vi "frontPanel.vi"(8 "error in (no error)":errorcluster, 10 "closeViewerEvent":refnum<user-event>, 11 "AnalysisResultsViewer in":refnum<class "AnalysisResultsViewer.lvclass">) -> (0 "error out":errorcluster, 3 "AnalysisResultsViewer out":refnum<class "AnalysisResultsViewer.lvclass">)   [LabVIEW 2009, in "Views.lvlib" / "Camera.lvlib" / "AnalysisResultsViewer.lvclass"]
uses:
  AnalysisResultsViewer.lvclass
  AnalysisResultsViewer.lvclass/AnalysisResultsViewer.ctl
panel:
  in  "timescale":dbl=1000.0
  in  "ResultsBox":i32(listbox)
  out "Cloud Size y":dbl(graph)
  in  "stop":bool
  out "Cloud Size x":dbl(graph)
  out "Atom Number":dbl(graph)
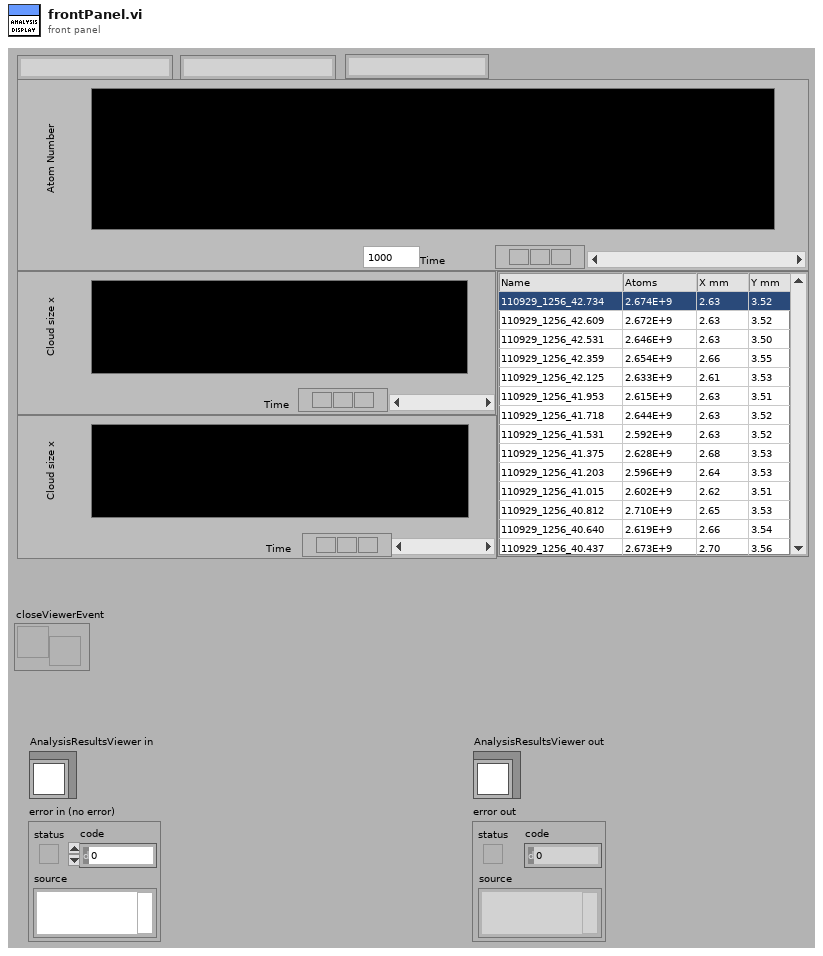
[diagram p1: front panel]
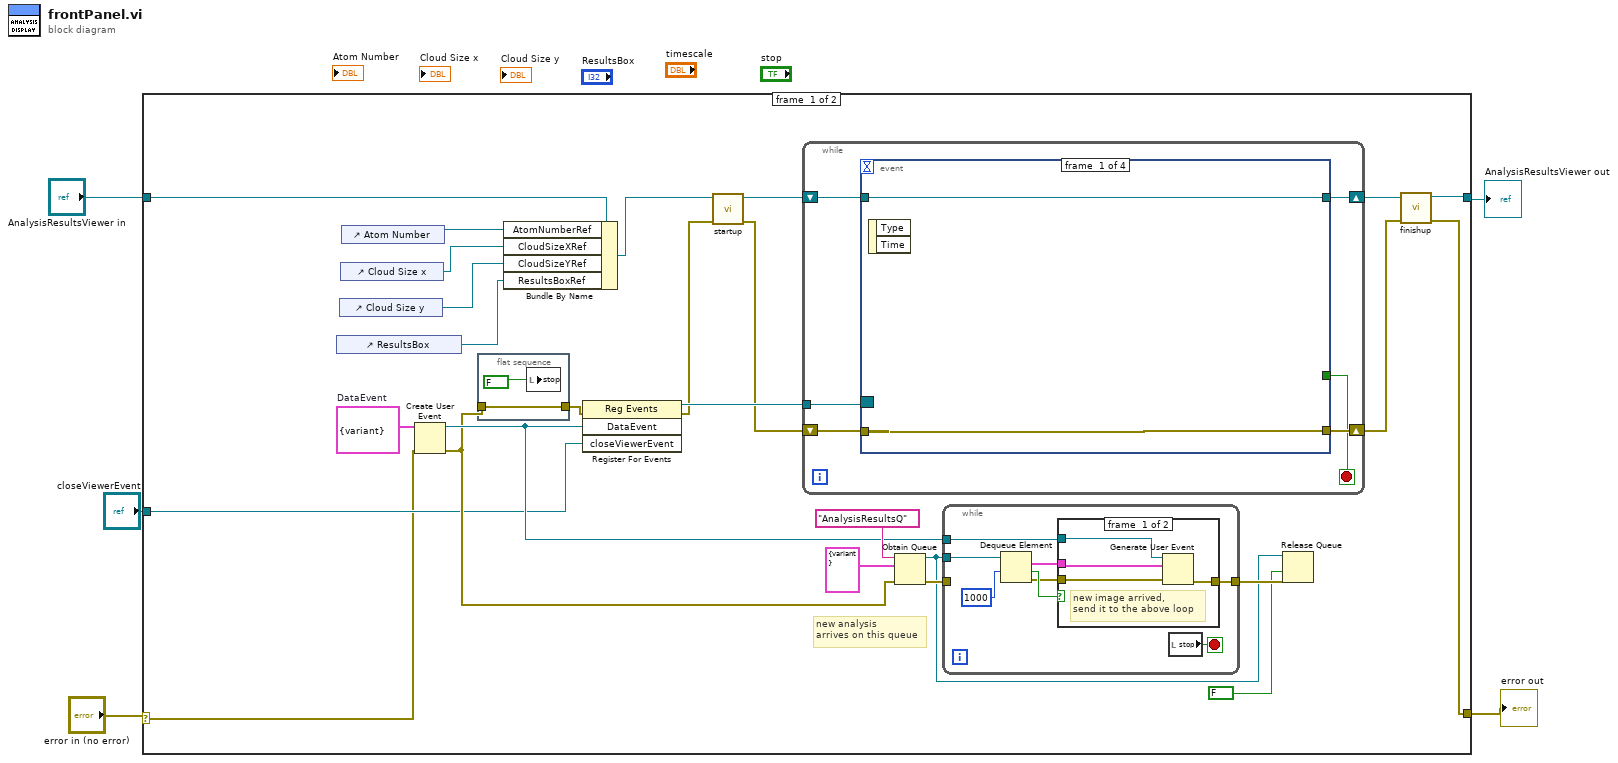
[diagram p0: block diagram]
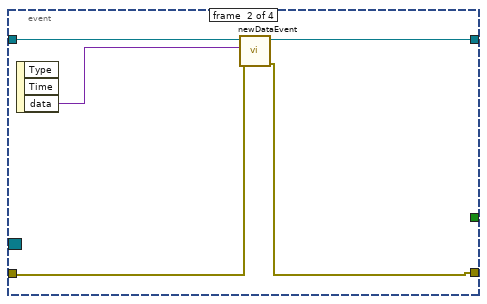
[diagram p3: hidden frame]
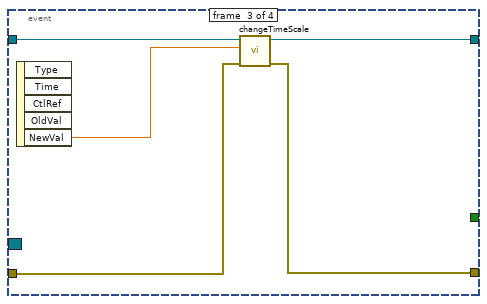
[diagram p4: hidden frame]
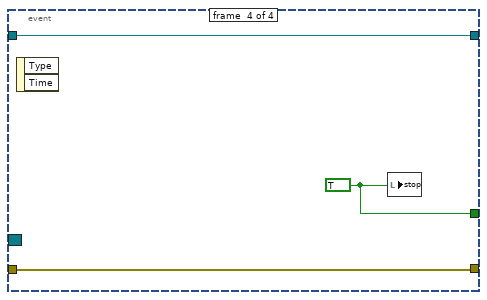
[diagram p5: hidden frame]
diagram:
  n1 = case shown="No Error" "error in (no error)" {
    selector: "error in (no error)" -> [w6 w69]
    tunnel: [w9 w69] -> w4
    tunnel: [w11 w68] -> w2
    tunnel: "AnalysisResultsViewer in" -> [w24 w68]
    tunnel: "closeViewerEvent" -> [w7 _]
    frame #0 {
      w26 = cluster{"data":variant} {"data"=variant}  # DataEvent
      # "new analysis\narrives on this queue"
      n2 = control-ref of="ResultsBox"() -> (w8:refnum<vi>)
      n3 = control-ref of="Cloud Size y"() -> (w21:refnum<vi>)
      n4 = control-ref of="Cloud Size x"() -> (w22:refnum<vi>)
      n5 = control-ref of="Atom Number"() -> (w23:refnum<vi>)
      n6 = Create User Event(user event datatype=w26, error in=w6) -> (user event=w18:refnum<user-event>, error out=w14:errorcluster)
      n7 = flat-sequence {
        tunnel: w14 -> [w33]
        tunnel: [w33] -> w13
        frame #0 {
          n8 = local write "stop"(FALSE) -> ()
        }
      }
      n9 = Bundle By Name(cluster=w24, "AtomNumberRef"=w23, "CloudSizeXRef"=w22, "CloudSizeYRef"=w21, "ResultsBoxRef"=w8) -> (w20:refnum<class "AnalysisResultsViewer.lvclass">)
      n10 = register-events(error in=w13, w18, w7) -> (reference out=w25:refnum<event-registration>, error out=w17:errorcluster)  [unwired: 1 in]
      n11 = call-dynamic "startup.vi"("error in (no error)"=w17, "AnalysisResultsViewer in"=w20) -> ("error out"=w16:errorcluster, "AnalysisResultsViewer out"=w19:refnum<class "AnalysisResultsViewer.lvclass">)  [unwired: 8 in]
      n12 = while {
        shift-right: [w52] -> w12
        shift-left: w19 -> [w51]
        tunnel: w25 -> [w50]
        shift-right: [w48] -> w10
        shift-left: w16 -> [w49]
        stop <- w47 stop-if-true
        n13 = event shown="[3] \"stop\": Mouse Down;  Panel Close;  <closeViewerEvent>: User Event" {
          selector: w50 -> [_ _ _ _]
          dyn-events: _ -> [_ _ _ _]
          timeout: _ -> [_ _ _ _]
          tunnel: [w54 w58 w63 w66] -> w52
          tunnel: w51 -> [w54 w59 w64 w66]
          tunnel: w49 -> [w53 w56 w61 w67]
          tunnel: [w53 w55 w60 w67] -> w48
          tunnel: [_ _ _ w65] -> w47
          event #0 {
            n14 = event-data() -> ()  [unwired: 1 in, 2 out]
          }
          event #1 {
            n15 = event-data() -> ("data"=w57:variant)  [unwired: 1 in, 2 out]
            n16 = call-dynamic "newDataEvent.vi"("error in (no error)"=w56, "data"=w57, "AnalysisResultsViewer in"=w59) -> ("error out"=w55:errorcluster, "AnalysisResultsViewer out"=w58:refnum<class "AnalysisResultsViewer.lvclass">)  [unwired: 7 in]
          }
          event #2 {
            n17 = event-data() -> ("NewVal"=w62:dbl)  [unwired: 1 in, 4 out]
            n18 = call "changeTimeScale.vi"("error in (no error)"=w61, "timescale"=w62, "AnalysisResultsViewer in"=w64) -> ("error out"=w60:errorcluster, "AnalysisResultsViewer out"=w63:refnum<class "AnalysisResultsViewer.lvclass">)  [unwired: 7 in]
          }
          event #3 {
            w65 = TRUE
            n19 = event-data() -> ()  [unwired: 1 in, 2 out]
            n20 = local write "stop"(w65) -> ()
          }
        }
      }
      n21 = Obtain Queue(name (unnamed)="AnalysisResultsQ", element data type=cluster{"data":variant} {"data"=variant} ("dataQ"), error in (no error)=w14) -> (queue out=w28:refnum<queue>, error out=w30:errorcluster)  [unwired: 2 in, 1 out]
      n22 = while {
        tunnel: w18 -> [w37]
        tunnel: w28 -> [w41]
        tunnel: w30 -> [_]
        tunnel: [w36] -> w29
        stop <- w35 stop-if-true
        n23 = Dequeue Element(queue=w41, timeout in ms (-1)=1000) -> (element=w34:cluster{"data":variant}, timed out?=w39:bool, error out=w38:errorcluster)  [unwired: 1 in, 1 out]
        n24 = case shown="False" w39 {
          tunnel: w38 -> [w45 w46]
          tunnel: w37 -> [w42 _]
          tunnel: [w44 w46] -> w36
          tunnel: w34 -> [w43 _]
          frame #0 {
            # "new image arrived, \nsend it to the above loop"
            n25 = Generate User Event(user event=w42, event data cluster=w43, error in=w45) -> (error out=w44:errorcluster)  [unwired: 1 out]
          }
          frame #1 {
            # "timeout"
          }
        }
        n26 = local read "stop"() -> (w35:bool)
      }
      n27 = Release Queue(queue=w28, force destroy? (F)=FALSE, error in (no error)=w29) -> ()  [unwired: 3 out]
      n28 = call-dynamic "finishup.vi"("error in (no error)"=w10, "AnalysisResultsViewer in"=w12) -> ("error out"=w9:errorcluster, "AnalysisResultsViewer out"=w11:refnum<class "AnalysisResultsViewer.lvclass">)  [unwired: 8 in]
    }
    frame #1 {
    }
  }
  "error out" <- w4
  "AnalysisResultsViewer out" <- w2
